vi "main_test.vi"() -> ()   [LabVIEW 2017]
panel:
  in  "vi path":path
  in  "stop":bool
  in  "Tab Control":enum32{"Page 1", "Page 2"}(tab)
  out "XY Graph":cluster{"all rows":dbl[], "all rows":dbl[]}[](graph)
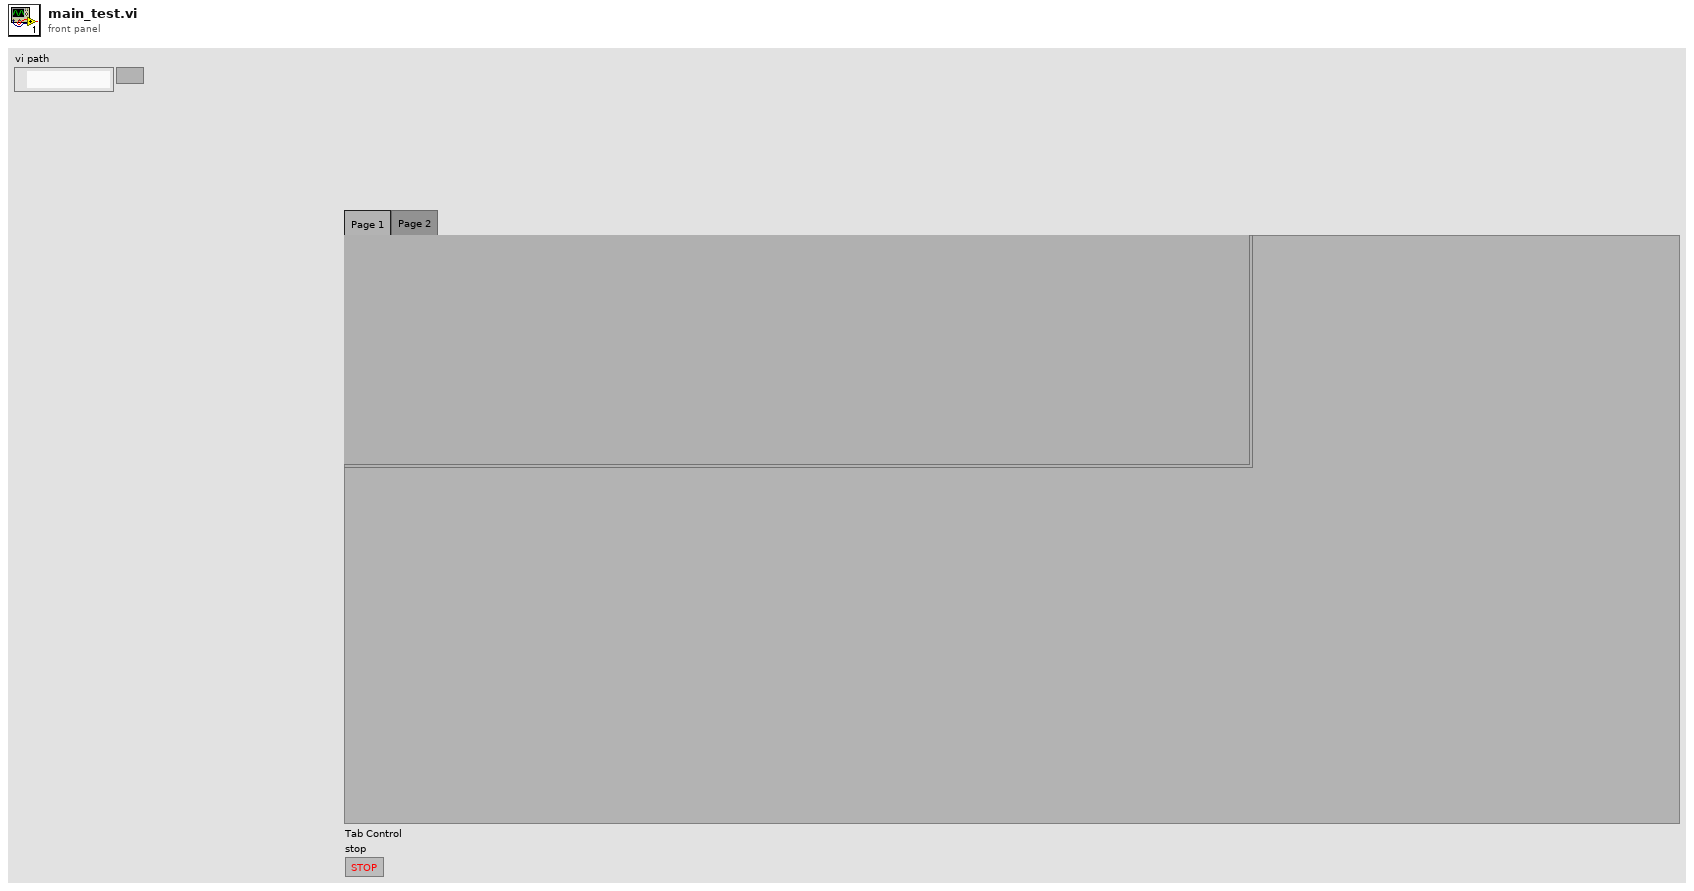
[diagram p1: front panel]
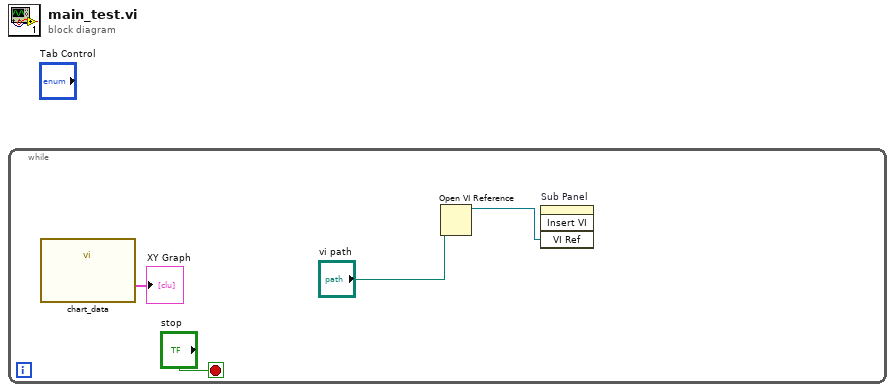
[diagram p0: block diagram]
diagram:
  n1 = while {
    stop <- "stop" stop-if-true
    n2 = call "chart_data.vi"() -> ("Output Graphs"=→"XY Graph":cluster{"all rows":dbl[], "all rows":dbl[]}[])  [unwired: 11 in]
    n3 = Open VI Reference(vi path="vi path") -> (vi reference=w2:refnum<vi>)  [unwired: 5 in, 1 out]
    n4 = invoke on="Sub Panel" class="SubPnl" method="Insert VI"("VI Ref"=w2) -> ()  [unwired: 3 in, 4 out]
  }
